vi "SRS_QCM_SubVI  dec2016.vi"(0 "VISA Refnum in":refnum<visa-resource-name>, 1 "first iteration?":bool, 5 "Frequency  in":dbl, 7 "SRS on?":bool, 9 "Gate time":u16(ring)=1 items=["0.1 seconds", "1.0 seconds", "10.0 seconds"], 11 "error in (no error)":errorcluster) -> (3 "Frequency out 2":dbl, 4 "freq, mass, MR":T1, 6 "Frequency out":dbl format="%#_8g", 8 "address out":T3, 10 "M":string, 13 "MR":string, 14 "F":string, 15 "M,F,MR output cluster":T2)   [LabVIEW 2014]
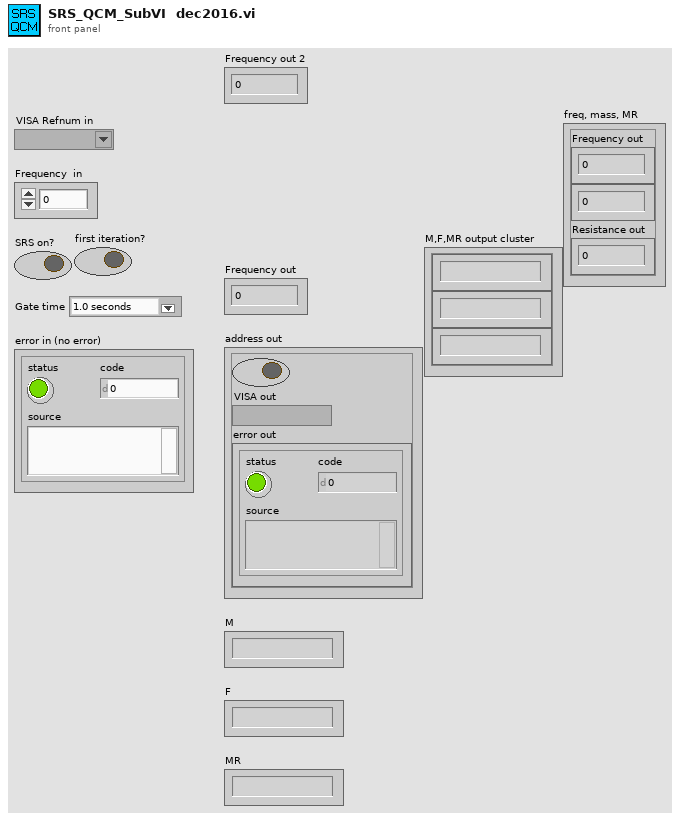
[diagram p1: front panel]
types:
  T1 = cluster{"Frequency out":dbl, "Numeric Control":dbl, "Resistance out":dbl}
  T2 = cluster{"String":string, "String":string, "String":string}
  T3 = cluster{"Boolean":bool, "VISA out":refnum<visa-resource-name>, "error out":errorcluster}
  T4 = cluster{"SRS on?":bool, "VISA out":refnum<visa-resource-name>, "error out":errorcluster}
  T5 = cluster{dbl, "Frequency out":dbl, "Resistance out":dbl}
  T6 = cluster{"Frequency out":dbl, dbl, "Resistance out":dbl}
  T7 = cluster{string, "Frequency out":string, "Resistance out":string}
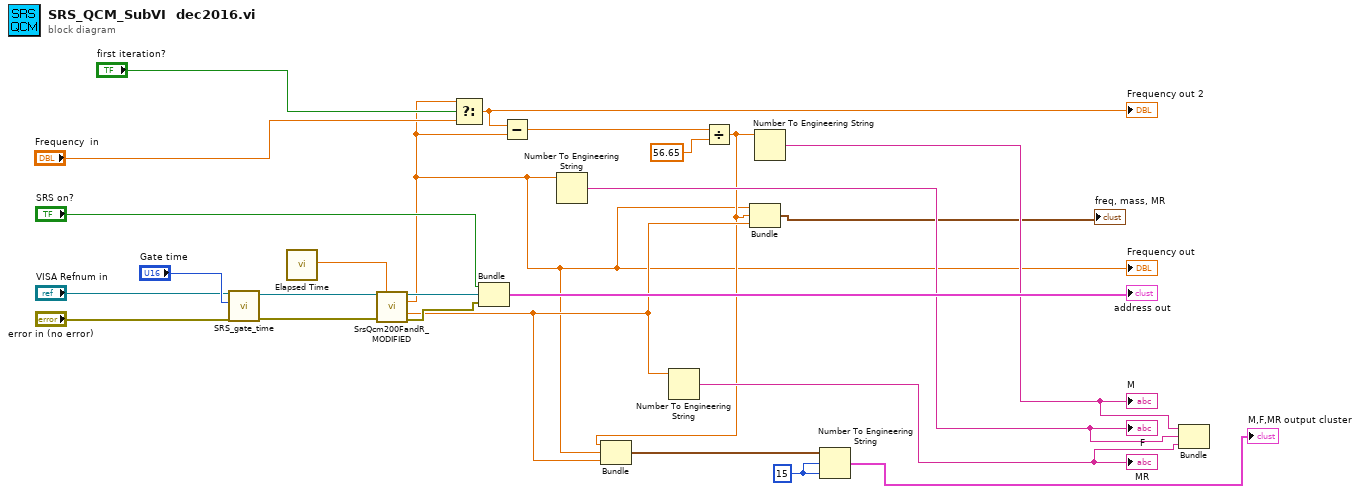
[diagram p0: block diagram]
diagram:
  w4 = i16 15 ("width (-)")
  n1 = call "SRS_gate_time.vi"("error in"="error in (no error)", "Gate time"="Gate time", "VISA in"="VISA Refnum in") -> ("error out"=w24:errorcluster, "VISA out"=w23:refnum<visa-resource-name>)  [unwired: 7 in]
  n2 = call "Elapsed Time"() -> ("Elapsed Time (s)"=w14:dbl)  [unwired: 12 in, 7 out]
  n3 = call "SrsQcm200FandR_MODIFIED.vi"("VISA in"=w23, "Reference time in"=w14, "error in (no error)"=w24) -> ("VISA out"=w16:refnum<visa-resource-name>, "Frequency out"=w2:dbl, "Resistance out"=w7:dbl, "error out"=w15:errorcluster)  [unwired: 6 in, 3 out]
  "Frequency out" <- w2
  n4 = Select(t=w2, s="first iteration?", f="Frequency  in") -> (s? t:f=w20:dbl)
  "Frequency out 2" <- w20
  n5 = Bundle("SRS on?"="SRS on?", "VISA out"=w16, "error out"=w15) -> (→"address out":T4)  [unwired: 1 in]
  n6 = Subtract(x=w20, y=w2) -> (x-y=w18:dbl)
  n7 = Number To Engineering String(4:w2) -> (0:w8:string)  [unwired: 3 in]
  "F" <- w8
  n8 = Number To Engineering String(4:w7) -> (0:w9:string)  [unwired: 3 in]
  "MR" <- w9
  n9 = Divide(x=w18, y=56.65) -> (x/y=w3:dbl)
  n10 = Bundle(w3, "Frequency out"=w2, "Resistance out"=w7) -> (w6:T5)  [unwired: 1 in]
  n11 = Bundle("Frequency out"=w2, w3, "Resistance out"=w7) -> (→"freq, mass, MR":T6)  [unwired: 1 in]
  n12 = Number To Engineering String(4:w3) -> (0:w10:string)  [unwired: 3 in]
  "M" <- w10
  n13 = Number To Engineering String(2:w4, 3:w4, 4:w6) -> (0:→"M,F,MR output cluster":T7)  [unwired: 1 in]
  n14 = Bundle(w10, w8, w9) -> ()  [unwired: 1 in, 1 out]
